vi "PSCMD_Toolbar Command.vi"(8 "error in":errorcluster, 10 "Data":variant, 11 "Command":T1) -> (0 "error out":errorcluster)   [LabVIEW 2016]
uses:
  DAQ Actor/API/PSDAQEG_Commoand Type.ctl
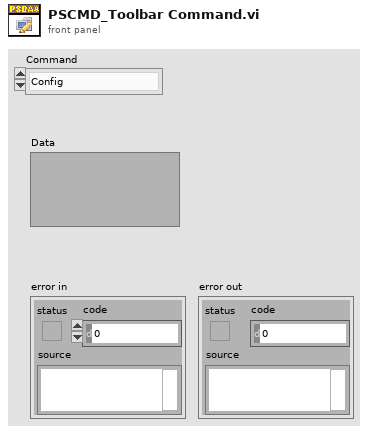
[diagram p1: front panel]
types:
  T1 = typedef "PSDAQEG_Commoand Type.ctl" = enum16{"Config", "Run", "Pause", "Stop", "Save"}
  T2 = cluster{"Main Queue":string, "DAQ Queue":string, "ANA Queue":string, "CUI Queue":string, "DRP Queue":string, "Graph Queue":string, "DOM Queue":string, "ACQ Queue":string, "MOD Queue":string, "OAA Queue":string, "REG Queue":string, "DRV Queue":string, "GEF Queue":string, "OVV Queue":string}
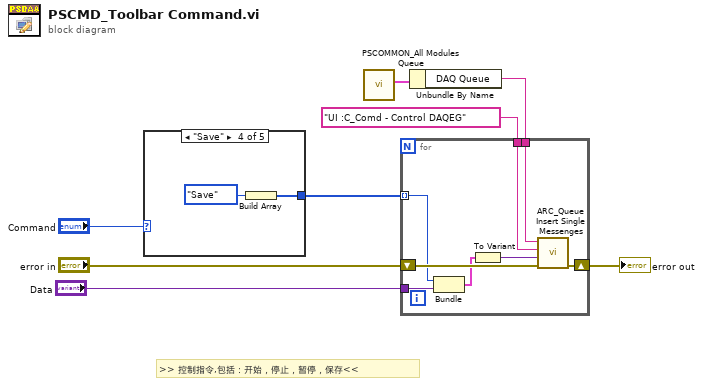
[diagram p0: block diagram]
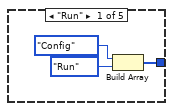
[diagram p2: hidden frame]
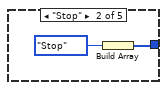
[diagram p3: hidden frame]
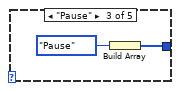
[diagram p4: hidden frame]
diagram:
  # ">> 控制指令,包括：开始，停止，暂停，保存<<"
  n1 = case shown="\"Save\"" "Command" {
    tunnel: [w11 w13 w15 w17 _] -> w8
    frame "Run" {
      n2 = Build Array(PSDAQEG_Commoand_Type."Config" ("Command"), PSDAQEG_Commoand_Type."Run" ("Command")) -> (w11:T1[])
    }
    frame "Stop" {
      n3 = Build Array(PSDAQEG_Commoand_Type."Stop" ("Command")) -> (w13:T1[])
    }
    frame "Pause" {
      n4 = Build Array(PSDAQEG_Commoand_Type."Pause" ("Command")) -> (w15:T1[])
    }
    frame "Save" {
      n5 = Build Array(PSDAQEG_Commoand_Type."Save" ("Command")) -> (w17:T1[])
    }
    frame "Config" {
    }
  }
  n6 = call "PSCOMMON_All Modules Queue.vi"() -> ("All Queues"=w2:T2)  [unwired: 11 in]
  n7 = Unbundle By Name(w2) -> ("DAQ Queue"=w1:string)
  n8 = for {
    tunnel: "UI :C_Comd - Control DAQEG" -> [w23]
    tunnel: w1 -> [w22]
    shift-right: [w24] -> w4
    shift-left: "error in" -> [w25]
    tunnel: w8 -> [w19] mode=indexing
    tunnel: "Data" -> [w20]
    n9 = Bundle("Command"=w19, "Data"=w20) -> (w18:cluster{"Command":T1, "Data":variant})  [unwired: 1 in]
    n10 = To Variant(anything=w18) -> (Variant=w21:variant)
    n11 = call "ARC_Queue Insert Single Messenges.vi"("error in (no error)"=w25, "Data"=w21, "Order"=w23, "Queue Name"=w22) -> ("error out"=w24:errorcluster)  [unwired: 7 in]
  }
  "error out" <- w4
